vi "Zero waveform.vi"(0 "reference in":refnum<class "Fcurve.lvclass">, 2 "Zero type":T3, 5 "error in (no error)":errorcluster) -> (8 "Def[0]":dbl, 10 "Zpos[0]":dbl, 14 "reference out":refnum<class "Fcurve.lvclass">, 16 "Zero Fcurve Segments":cluster{"X":dbl[], "Y":dbl[]}[](array[cluster]), 19 "error out":errorcluster)   [LabVIEW 2019, in "Fcurve.lvclass"]
doc: "Gets the first value of the index and subtracts it from the rest."
uses:
  Fcurve.lvclass
  Zero Type.ctl
  <vilib>/Analysis/6fits.llb/Curve Fitting Criteria.ctl
  metadata_class/Segment type--combobox.ctl
  <vilib>/Analysis/NI_AALPro.lvlib
  metadata_class/metadata.lvclass
  <vilib>/Analysis/NI_AALBase.lvlib
panel:
  out "variance":dbl format="%0.2f"
  out "standard deviation":dbl format="%0.2f"
  out "mean":dbl format="%0.2f"
  out "intercept":dbl
  out "slope":dbl
  in  "method":T1 items=["Least Square", "Least Absolute Residual", "Bisquare"]
  in  "parameter bounds":T2={"slope min"=-inf, "slope max"=inf, "intercept min"=-inf, "intercept max"=inf}
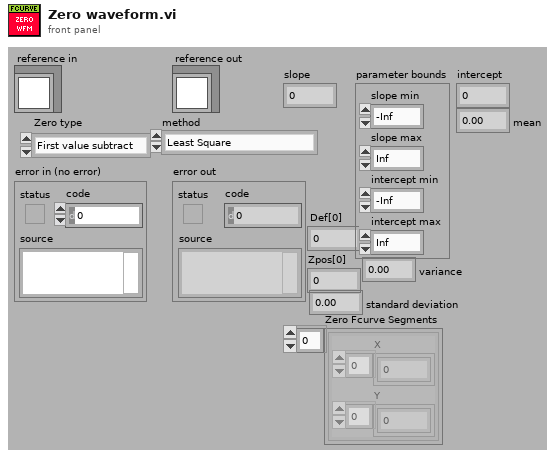
[diagram p1: front panel]
types:
  T1 = typedef "NI_AALPro.lvlib/Curve Fitting Criteria.ctl" = u16
  T2 = cluster{"slope min":dbl, "slope max":dbl, "intercept min":dbl, "intercept max":dbl}
  T3 = typedef "Fcurve.lvclass/Zero Type.ctl" = enum16{"First value subtract", "Median (approach)", "Linear fit (approach)"}
  T4 = typedef "metadata.lvclass/Segment type--combobox.ctl" = string
  T5 = typedef "Fcurve.lvclass/ObjectAttributesRef.ctl" = refnum<data-value>
  T6 = typedef "Fcurve.lvclass/ObjectAttributes.ctl" = cluster{"MyAttribute":dbl, "Fcurve Metadata":T7, "Contact Spread of dev":dbl, "Tau Delay (ms)":dbl, "Points of contact":dbl, "Def_wfm":cluster{"Max":dbl, "Min":dbl}, "Zpos_wfm":cluster{"Max":dbl, "Min":dbl}, "Contact stat?":bool, "Real AI dt (s)":dbl, "Decimation":cluster{"App":cluster{"Dec":i32, "apply":bool}, "Con":cluster{"Dec":i32, "apply":bool}, "Ret":cluster{"Dec":i32, "apply":bool}}, "Segment def[0]":dbl, "Segment Zpos[0]":dbl, "Raw Datum":waveform(dbl)[], "Group metadata":T8, "M_data obj":refnum<class "metadata.lvclass">, "Channel name(s)":string[], "Segment fcurve data":cluster{"X":dbl[], "Y":dbl[]}[], "Segment duration":cluster{"Start":i32, "Duration":i32}[], "Segment info":T9[], "Segment durations (S)":dbl[], "Segments Maxmin":T10[]}
  T7 = typedef "Fcurve.lvclass/Metadata.ctl" = cluster{"dt (us)":dbl, "Dec Factor":dbl, "Z piezo Sensitivity (nm/V)":dbl, "K (N/m)":dbl, "Sp (V)":dbl, "Contact (ms)":dbl, "Zpos contact":dbl, "Vel_app (nm/s)":dbl, "Vel_ret (nm/s)":dbl, "deltaV (nm)":dbl, "Def_V0 (v)":dbl, "Piezo gain":dbl, "invOLS (nm/V)":dbl}
  T8 = typedef "TDMS_DataHandler.lvclass/Fcurve Meta data.ctl" = cluster{"property names":string[], "property values":variant[]}
  T9 = typedef "Fcurve.lvclass/Fcurve segments --cluster.ctl" = cluster{"type":T4, "nb points":i32, "dec factor":u32, "sampling rate (S/s)":u32}
  T10 = typedef "Fcurve.lvclass/Segment MaxMin --cluster.ctl" = cluster{"Def":cluster{"max value":dbl, "min value":dbl}, "Zpos":cluster{"max value":dbl, "min value":dbl}}
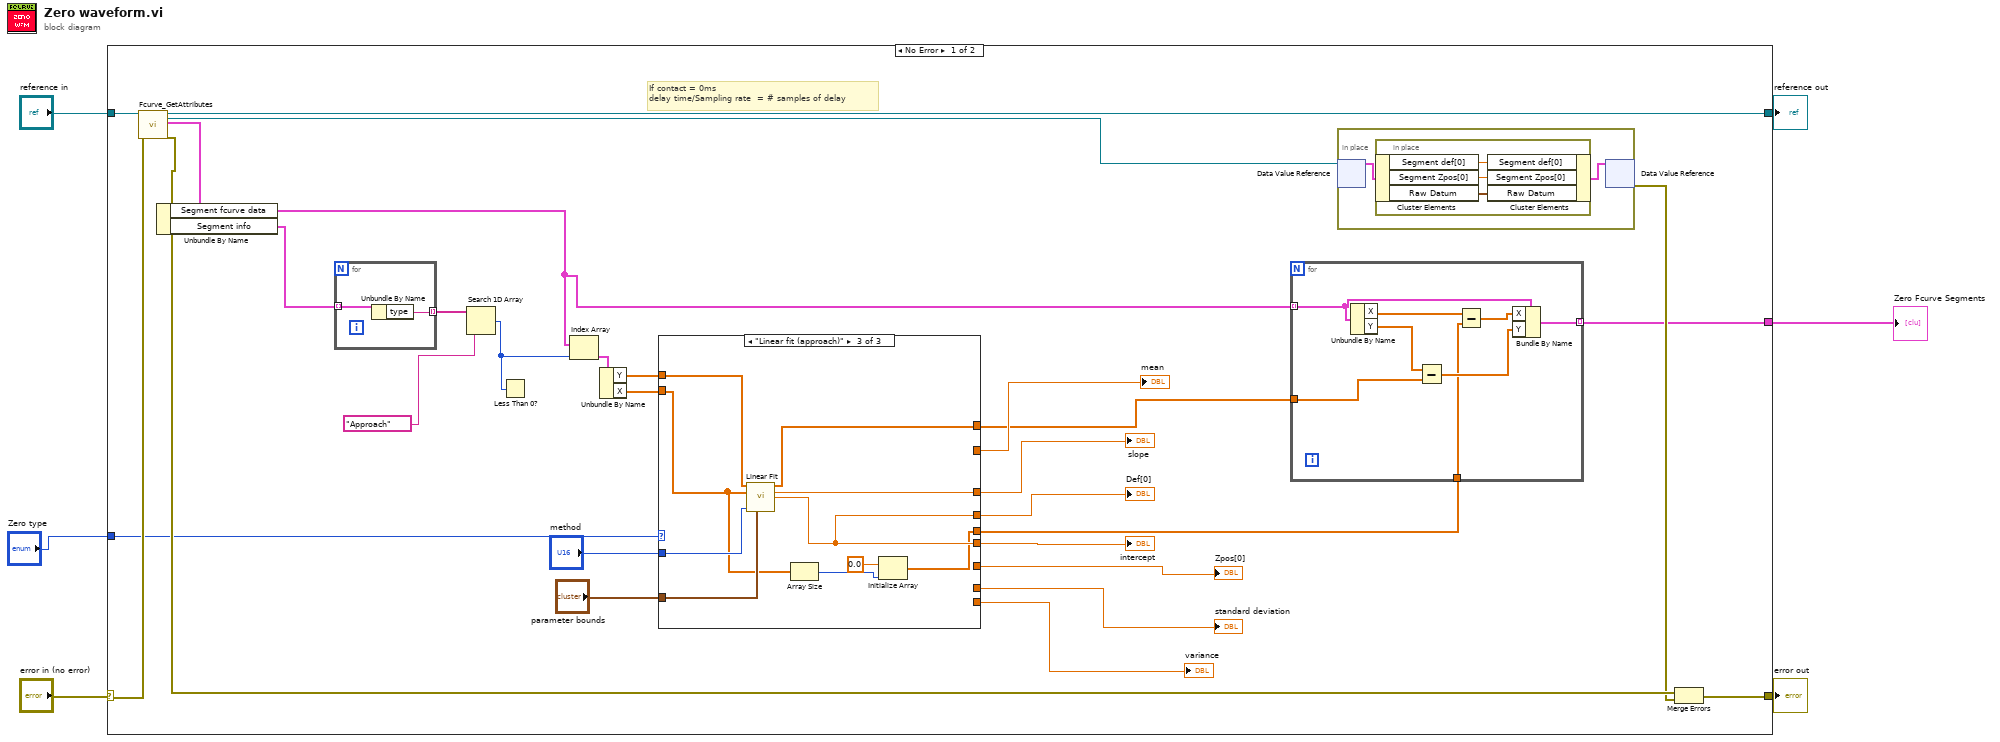
[diagram p0: block diagram]
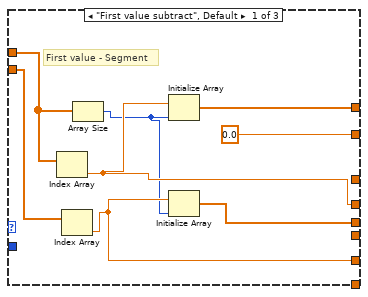
[diagram p2: hidden frame]
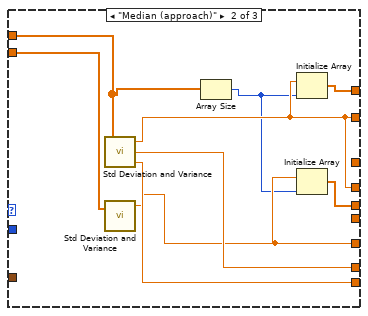
[diagram p3: hidden frame]
diagram:
  n1 = case shown="No Error" "error in (no error)" {
    selector: "error in (no error)" -> [w33 w79]
    tunnel: [w35 w79] -> w5
    tunnel: [w34 w78] -> w3
    tunnel: "reference in" -> [w32 w78]
    tunnel: "Zero type" -> [w27 _]
    tunnel: [w10 _] -> w1
    frame No Error {
      # "If contact = 0ms\ndelay time/Sampling rate  = # samples of delay"
      n2 = call "Fcurve_GetAttributes.vi"("reference in"=w32, "error in (no error)"=w33) -> ("reference out"=w34:refnum<class "Fcurve.lvclass">, "attributes ref"=w29:T5, "attributes"=w28:T6, "error out"=w31:errorcluster)  [unwired: 14 in]
      n3 = Unbundle By Name(w28) -> ("Segment fcurve data"=w13:cluster{"X":dbl[], "Y":dbl[]}[], "Segment info"=w24:T9[])
      n4 = for {
        tunnel: w24 -> [w45] mode=indexing
        tunnel: [w44] -> w23 mode=indexing
        n5 = Unbundle By Name(w45) -> ("type"=w44:T4)
      }
      n6 = Search 1D Array(1D array=w23, element=T4 "Approach" ("type")) -> (index of element=w22:i32)  [unwired: 1 in]
      n7 = Less Than 0?(x=w22) -> ()  [unwired: 1 out]
      n8 = Index Array(array=w13, index=w22) -> (element=w14:cluster{"X":dbl[], "Y":dbl[]})
      n9 = Unbundle By Name(w14) -> ("Y"=w25:dbl[], "X"=w26:dbl[])
      n10 = case shown="\"Linear fit (approach)\"" w27 {
        tunnel: w26 -> [w53 w60 w66]
        tunnel: w25 -> [w50 w55 w69]
        tunnel: "parameter bounds" -> [_ _ w72]
        tunnel: "method" -> [_ _ w71]
        tunnel: [_ _ w70] -> w19
        tunnel: [_ _ w68] -> w18
        tunnel: [0.0 ("mean") w59 _] -> w17
        tunnel: [_ w62 _] -> w16
        tunnel: [_ w61 _] -> w15
        tunnel: [w51 w59 w68] -> w12
        tunnel: [w48 w57 _] -> w11
        tunnel: [w49 w58 w67] -> w8
        tunnel: [w46 w54 w63] -> w7
        frame "First value subtract", Default {
          # "First value - Segment"
          n11 = Index Array(array=w50) -> (element=w51:dbl)  [unwired: 1 in]
          n12 = Index Array(array=w53) -> (element=w48:dbl)  [unwired: 1 in]
          n13 = Array Size(array=w50) -> (size(s)=w47:i32)
          n14 = Initialize Array(w51, w47) -> (w49:dbl[])
          n15 = Initialize Array(w48, w47) -> (w46:dbl[])
        }
        frame "Median (approach)" {
          n16 = call <vilib>:"Std Deviation and Variance.vi"("X"=w55) -> ("mean"=w59:dbl, "standard deviation"=w62:dbl, "variance"=w61:dbl)  [unwired: 1 in]
          n17 = call <vilib>:"Std Deviation and Variance.vi"("X"=w60) -> ("mean"=w57:dbl)  [unwired: 1 in, 2 out]
          n18 = Array Size(array=w55) -> (size(s)=w56:i32)
          n19 = Initialize Array(w59, w56) -> (w58:dbl[])
          n20 = Initialize Array(w57, w56) -> (w54:dbl[])
        }
        frame "Linear fit (approach)" {
          n21 = call <vilib>:"Linear Fit.vi"("Y"=w69, "X"=w66, "method"=w71, "parameter bounds"=w72) -> ("Best Linear Fit"=w67:dbl[], "slope"=w70:dbl, "intercept"=w68:dbl)  [unwired: 7 in, 2 out]
          n22 = Array Size(array=w66) -> (size(s)=w65:i32)
          n23 = Initialize Array(0.0 ("element"), w65) -> (w63:dbl[])
        }
      }
      "Def[0]" <- w12
      "Zpos[0]" <- w11
      "slope" <- w19
      "intercept" <- w18
      "mean" <- w17
      "standard deviation" <- w16
      "variance" <- w15
      n24 = for {
        tunnel: w13 -> [w42] mode=indexing
        tunnel: [w40] -> w10 mode=indexing
        tunnel: w8 -> [w37]
        tunnel: w7 -> [w36]
        n25 = Unbundle By Name(w42) -> ("X"=w41:dbl[], "Y"=w43:dbl[])
        n26 = Subtract(x=w43, y=w37) -> (x-y=w38:dbl[])
        n27 = Subtract(x=w41, y=w36) -> (x-y=w39:dbl[])
        n28 = Bundle By Name(cluster=w42, "X"=w39, "Y"=w38) -> (w40:cluster{"X":dbl[], "Y":dbl[]})
      }
      n29 = in-place {
        n30 = in-place-dvr #1(w29) -> (w73:T6)  [unwired: 1 out]
        n31 = in-place {
          n32 = in-place-cluster #2(w73) -> ("Segment def[0]"=w77:dbl, "Segment Zpos[0]"=w76:dbl, "Raw Datum"=w75:waveform(dbl)[])
          n33 = in-place-cluster #2("Segment def[0]"=w77, "Segment Zpos[0]"=w76, "Raw Datum"=w75) -> (w74:T6)
        }
        n34 = in-place-dvr #1(w74) -> (w30:errorcluster)  [unwired: 1 out]
      }
      n35 = Merge Errors(w31, w30) -> (w35:errorcluster)
    }
    frame Error {
    }
  }
  "error out" <- w5
  "reference out" <- w3
  "Zero Fcurve Segments" <- w1
